vi "BackupCode.vi"() -> ()   [LabVIEW 2012]
uses:
  Status.ctl
  StimulCtrls.lvlib
  SubPanels/InputPadRef.vi
  UserControl/ElectdTerminal.ctl
  UserControl/ElectdPanel.ctl
  UserControl/LeftPanel.ctl
  COR/CohortConfig.ctl
  UserControl/Cohort_sm.ctl
  SEQPool/SEQPool.ctl
panel:
  out "Pool":T1 {"Seed 8"."Delay Time" format="%.3f"; "Seed 7"."Delay Time" format="%.3f"; "Seed 6"."Delay Time" format="%.3f"; "Seed 5"."Delay Time" format="%.3f"; "Seed 4"."Delay Time" format="%.3f"; "Seed 3"."Delay Time" format="%.3f"; "Seed 2"."Delay Time" format="%.3f"; "Seed 1"."Delay Time" format="%.3f"; "Seed 0"."Delay Time" format="%.3f"}
  in  "Max SEQ":u8
  in  "Cohort Panel":T3={"Frequency [Hz]"=55.0, "Pulse Width [ms]"=194.0, "Basic Unit"={"Electrode"={"Group #"="", "T #"=0, "Magnitude"=0.0, "check"=FALSE}, "Electrode 2"={"Group #"="", "T #"=0, "Magnitude"=0.0, "check"=FALSE}, "Electrode 3"={"Group #"="", "T #"=0, "Magnitude"=0.0, "check"=FALSE}, "Electrode 4"={"Group #"="", "T #"=0, "Magnitude"=0.0, "check"=FALSE}, "Electrode 5"={"Group #"="", "T #"=0, "Magnitude"=0.0, "check"=FALSE}, "Electrode 6"={"Group #"="", "T #"=0, "Magnitude"=0.0, "check"=FALSE}, "Electrode 7"={"Group #"="", "T #"=0, "Magnitude"=0.0, "check"=FALSE}, "Electrode 8"={"Group #"="", "T #"=0, "Magnitude"=0.0, "check"=FALSE}, "Electrode 9"={"Group #"="", "T #"=0, "Magnitude"=0.0, "check"=FALSE}, "Electrode 10"={"Group #"="", "T #"=0, "Magnitude"=0.0, "check"=FALSE}, "Electrode 11"={"Group #"="", "T #"=0, "Magnitude"=0.0, "check"=FALSE}, "Electrode 12"={"Group #"="", "T #"=0, "Magnitude"=0.0, "check"=FALSE}, "Electrode 13"={"Group #"="", "T #"=0, "Magnitude"=0.0, "check"=FALSE}, "Electrode 14"={"Group #"="", "T #"=0, "Magnitude"=0.0, "check"=FALSE}, "Electrode 15"={"Group #"="", "T #"=0, "Magnitude"=0.0, "check"=FALSE}, "Electrode 16"={"Group #"="", "T #"=0, "Magnitude"=0.0, "check"=FALSE}}, "Tag"=""} {"Pulse Width [ms]" format="%#_6p"; "Basic Unit"."Electrode 16"."Magnitude" format="%4.2f"; "Basic Unit"."Electrode 15"."Magnitude" format="%4.2f"; "Basic Unit"."Electrode 14"."Magnitude" format="%4.2f"; "Basic Unit"."Electrode 13"."Magnitude" format="%4.2f"; "Basic Unit"."Electrode 12"."Magnitude" format="%4.2f"; "Basic Unit"."Electrode 11"."Magnitude" format="%4.2f"; "Basic Unit"."Electrode 10"."Magnitude" format="%4.2f"; "Basic Unit"."Electrode 9"."Magnitude" format="%4.2f"; "Basic Unit"."Electrode 8"."Magnitude" format="%4.2f"; "Basic Unit"."Electrode 7"."Magnitude" format="%4.2f"; "Basic Unit"."Electrode 6"."Magnitude" format="%4.2f"; "Basic Unit"."Electrode 5"."Magnitude" format="%4.2f"; "Basic Unit"."Electrode 4"."Magnitude" format="%4.2f"; "Basic Unit"."Electrode 3"."Magnitude" format="%4.2f"; "Basic Unit"."Electrode 2"."Magnitude" format="%4.2f"; "Basic Unit"."Electrode"."Magnitude" format="%4.2f"}
  in  "stop":bool
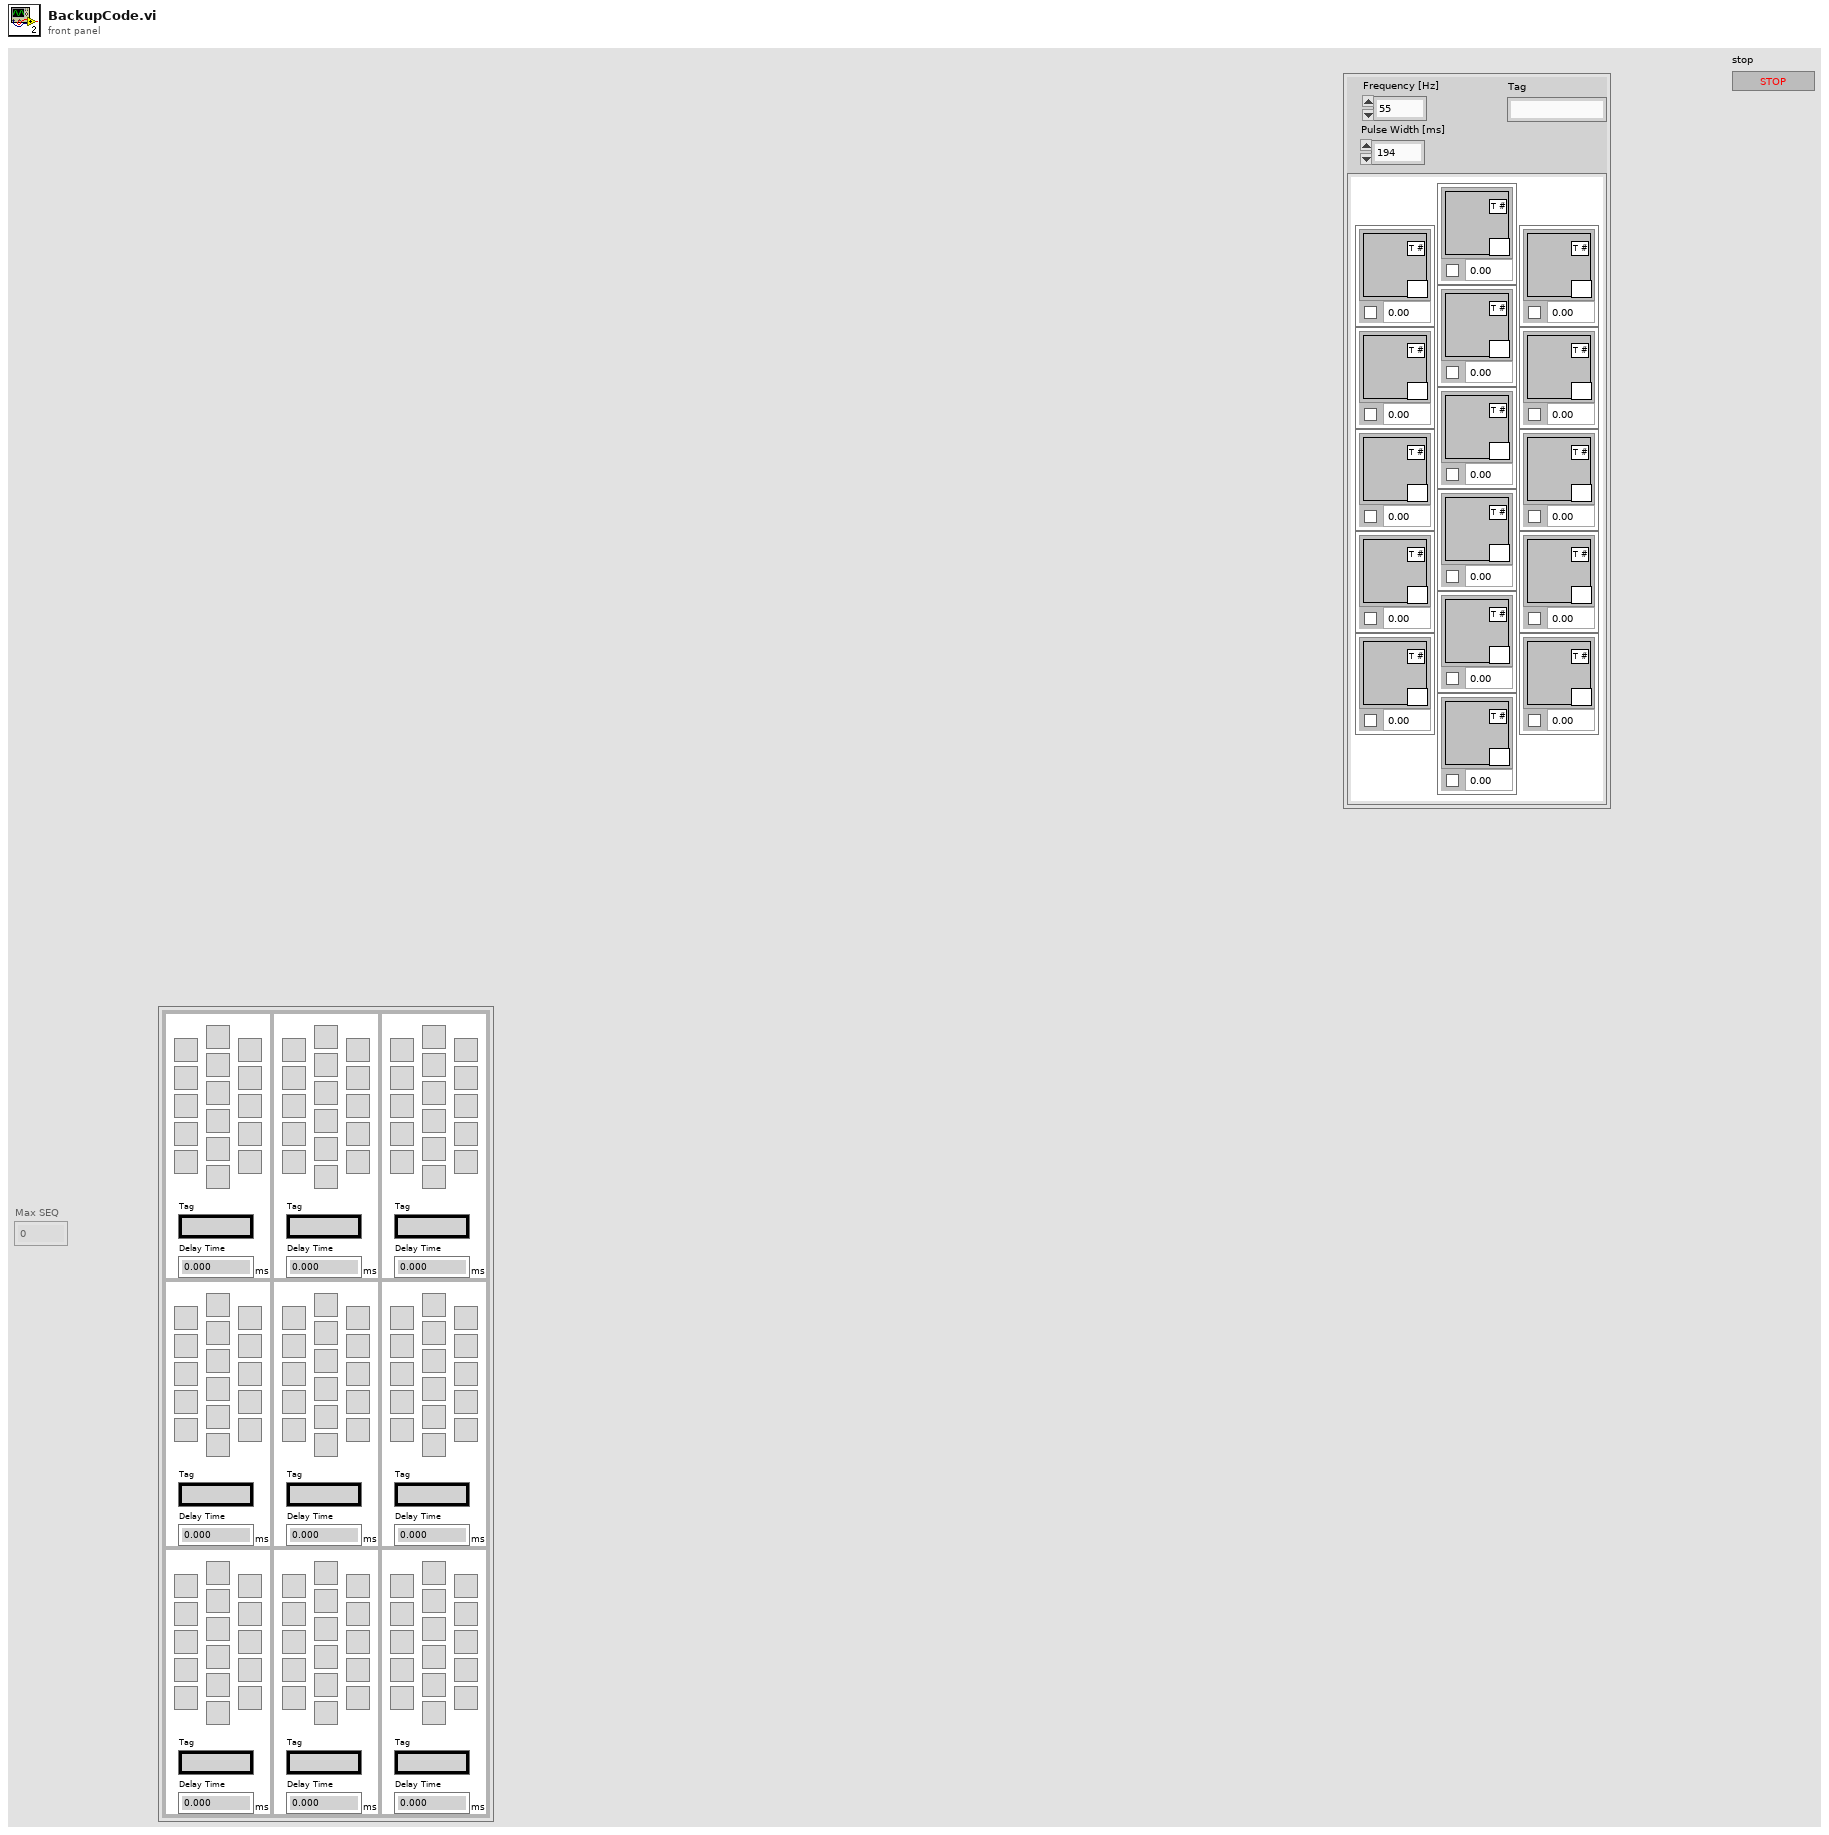
[diagram p1: front panel]
types:
  T1 = typedef "StimulCtrls.lvlib/SEQPool.ctl" = cluster{"Seed 0":T2, "Seed 1":T2, "Seed 2":T2, "Seed 3":T2, "Seed 4":T2, "Seed 5":T2, "Seed 6":T2, "Seed 7":T2, "Seed 8":T2}
  T2 = typedef "StimulCtrls.lvlib/Cohort_sm.ctl" = cluster{"Simplified Panel":cluster{"BU 0":cluster{"Electrode":u16}, "BU 1":cluster{"Electrode":u16}, "BU 2":cluster{"Electrode":u16}, "BU 3":cluster{"Electrode":u16}, "BU 4":cluster{"Electrode":u16}, "BU 5":cluster{"Electrode":u16}, "BU 6":cluster{"Electrode":u16}, "BU 7":cluster{"Electrode":u16}, "BU 8":cluster{"Electrode":u16}, "BU 9":cluster{"Electrode":u16}, "BU 10":cluster{"Electrode":u16}, "BU 11":cluster{"Electrode":u16}, "BU 12":cluster{"Electrode":u16}, "BU 13":cluster{"Electrode":u16}, "BU 14":cluster{"Electrode":u16}, "BU 15":cluster{"Electrode":u16}}, "Tag":string, "Delay Time":dbl[unit]}
  T3 = typedef "StimulCtrls.lvlib/CohortConfig.ctl" = cluster{"Frequency [Hz]":sgl, "Pulse Width [ms]":sgl, "Basic Unit":T4, "Tag":string}
  T4 = typedef "StimulCtrls.lvlib/LeftPanel.ctl" = cluster{"Electrode":T5, "Electrode 2":T5, "Electrode 3":T5, "Electrode 4":T5, "Electrode 5":T5, "Electrode 6":T5, "Electrode 7":T5, "Electrode 8":T5, "Electrode 9":T5, "Electrode 10":T5, "Electrode 11":T5, "Electrode 12":T5, "Electrode 13":T5, "Electrode 14":T5, "Electrode 15":T5, "Electrode 16":T5}
  T5 = typedef "StimulCtrls.lvlib/ElectdPanel.ctl" = cluster{"Group #":string, "T #":T6, "Magnitude":sgl, "check":bool}
  T6 = typedef "StimulCtrls.lvlib/ElectdTerminal.ctl" = u8
  T7 = typedef "StimulCtrls.lvlib/Status.ctl" = enum16{"SeqOpen", "CohortShow", "Wait", "Stop", "UpdateLeftPanel", "SeqSave", "CohortUpdate", "CohortAdd", "CohortClear", "CohortDel", "CohortBatch", "InputCall", "CohortCheck", "ProgQuit", "CohortQuickAmp", "CohortQuickState", "Initializing", "SeqCheck", "CylEdit", "PrgEdit", "PoolSelect"}
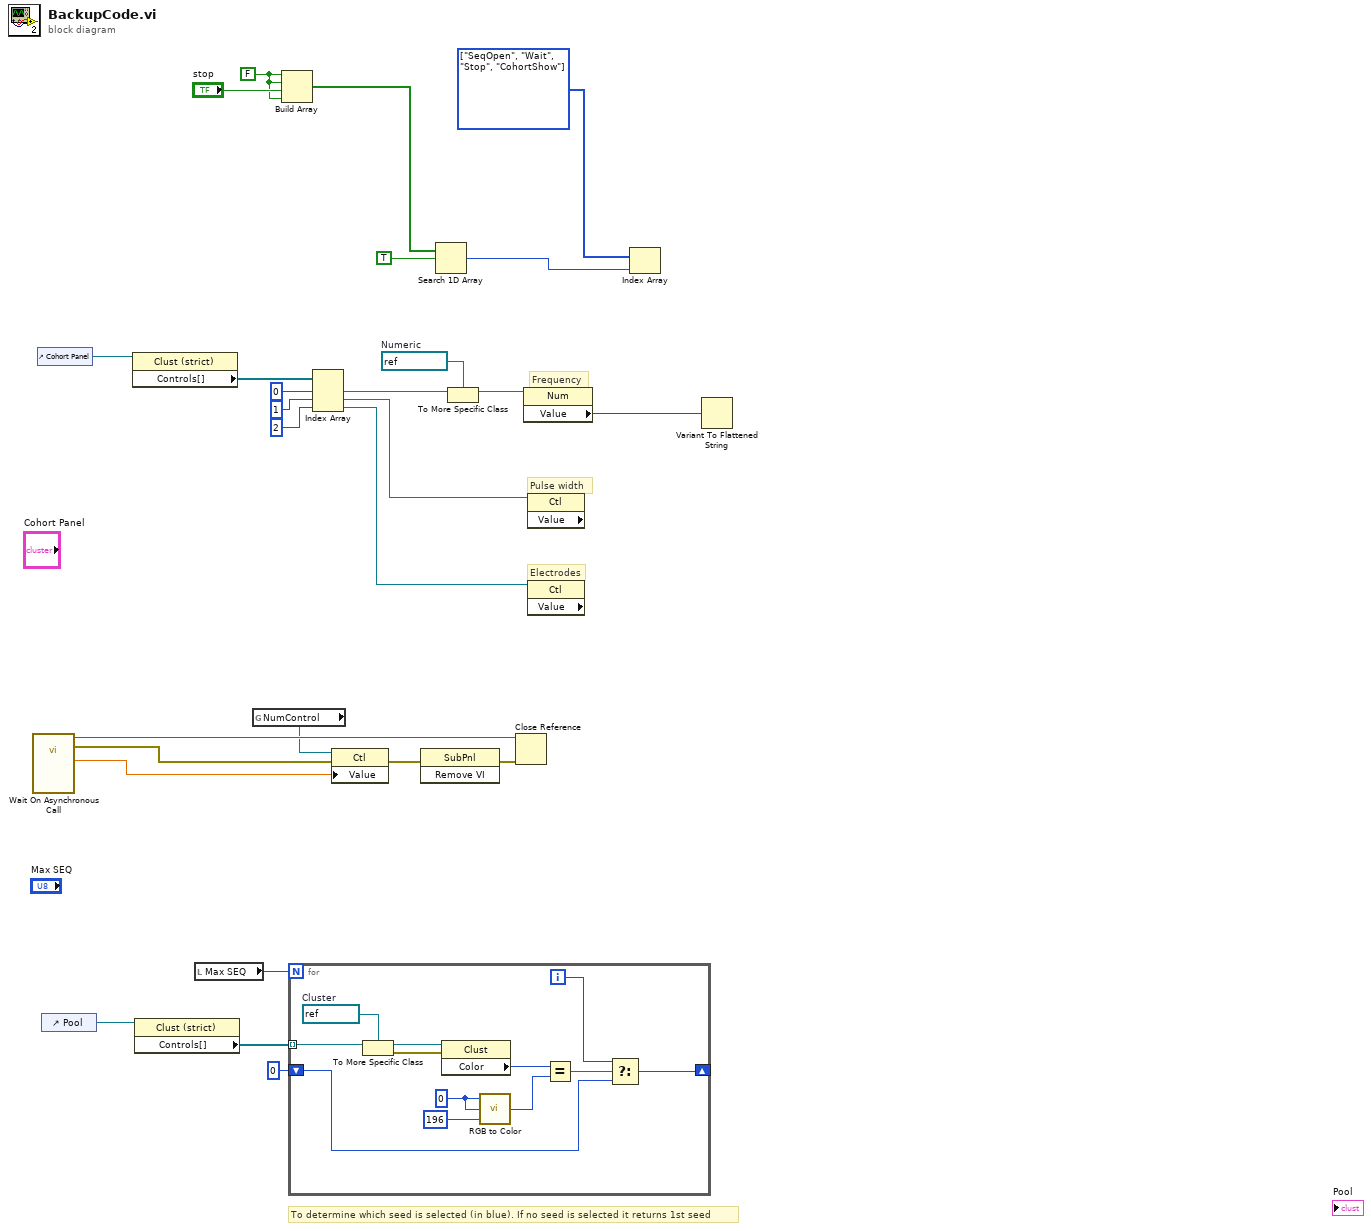
[diagram p0: block diagram]
diagram:
  w14 = refnum<vi> refnum  # Numeric
  w23 = FALSE
  w28 = T7[] [enum."SeqOpen", enum."Wait", enum."Stop", enum."CohortShow"] items=["SeqOpen", "CohortShow", "Wait", "Stop", "UpdateLeftPanel", "SeqSave", "CohortUpdate", "CohortAdd", "CohortClear", "CohortDel", "CohortBatch", "InputCall", "CohortCheck", "ProgQuit", "CohortQuickAmp", "CohortQuickState", "Initializing", "SeqCheck", "CylEdit", "PrgEdit", "PoolSelect"]
  # "To determine which seed is selected (in blue). If no seed is selected it returns 1st seed"
  # "Electrodes"
  # "Pulse width"
  # "Frequency"
  n1 = call-by-ref "Wait On Asynchronous Call"() -> (reference out=w9:refnum<vi>, error out=w11:errorcluster, "PadIndicator"=w10:dbl)  [unwired: 13 in]
  n2 = control-ref of="Cohort Panel"() -> (w22:refnum<vi>)
  n3 = control-ref of="Pool"() -> (w5:refnum<vi>)
  n4 = property class="Clust (strict)"(reference=w22) -> ("Controls[]"=w21:refnum<vi>[])  [unwired: 1 in, 2 out]
  n5 = property class="Clust (strict)"(reference=w5) -> ("Controls[]"=w4:refnum<vi>[])  [unwired: 1 in, 2 out]
  n6 = local read "Max SEQ"() -> (w1:u8)
  n7 = global read "InputPadRef.vi" "NumControl"() -> (w8:refnum<vi>)
  n8 = Build Array(w23, w23, "stop", w23) -> (w25:bool[])
  n9 = for {
    N: w1 -> [_]
    tunnel: w4 -> [w40] mode=indexing
    shift-right: [w30] -> w2
    shift-left: 0 -> [w29]
    i -> [w31]
    w36 = u8 0 ("R")
    w39 = refnum<vi> refnum  # Cluster
    n10 = To More Specific Class(target class=w39, reference=w40) -> (specific class reference=w38:refnum<vi>, error out=w37:errorcluster)  [unwired: 1 in]
    n11 = property class="Clust"(reference=w38, error in=w37) -> ("Color"=w34:u32)  [unwired: 2 out]
    n12 = call <vilib>:"RGB to Color.vi"("B"=u8 196, "G"=w36, "R"=w36) -> ("Color"=w33:u32)
    n13 = Equal?(x=w34, y=w33) -> (x = y?=w32:bool)
    n14 = Select(t=w31, s=w32, f=w29) -> (s? t:f=w30:i32)
  }
  n15 = Index Array(array=w21, index #1=0 ("index"), index #2=1 ("index"), index #3=2 ("index")) -> (element #1=w17:refnum<vi>, element #2=w16:refnum<vi>, element #3=w15:refnum<vi>)
  n16 = property class="Ctl"(reference=w8, error in=w11, "Value"=w10) -> (error out=w7:errorcluster)  [unwired: 1 out]
  n17 = invoke on="Invoke Node" class="SubPnl" method="Remove VI"(error in=w7) -> (error out=w6:errorcluster)  [unwired: 2 in, 2 out]
  n18 = Search 1D Array(1D array=w25, element=TRUE) -> (index of element=w24:i32)  [unwired: 1 in]
  n19 = To More Specific Class(target class=w14, reference=w17) -> (specific class reference=w13:refnum<vi>)  [unwired: 1 in, 1 out]
  n20 = Close Reference(reference=w9, error in (no error)=w6) -> ()  [unwired: 1 out]
  n21 = property class="Num"(reference=w13) -> ("Value"=w12:variant)  [unwired: 1 in, 2 out]
  n22 = property class="Ctl" props=["Value"](reference=w16) -> ()  [unwired: 1 in, 3 out]
  n23 = property class="Ctl" props=["Value"](reference=w15) -> ()  [unwired: 1 in, 3 out]
  n24 = Index Array(array=w28, index=w24) -> ()  [unwired: 1 out]
  n25 = Variant To Flattened String(Variant=w12) -> ()  [unwired: 2 out]
